vi "Word Find & Replace.vi"   [LabVIEW 2010, in "NI_ReportGenerationToolkit.lvlib"]
doc: "Finds and replaces a text segment. The data type you wire to the <B>replace with</B> input determines the polymorphic instance to use."
uses:
  <vilib>/addons/_office/NI_ReportGenerationToolkit.lvlib
  <vilib>/Utility/NIReport.llb/Word/NI_Word.lvclass
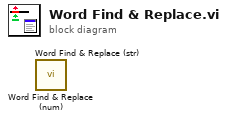
[diagram p0: block diagram]
diagram:
  n1 = call <vilib>:"Word Find & Replace (num).vi"() -> ()  [unwired: 13 in, 3 out]
  n2 = call "Word Find & Replace (str).vi"() -> ()  [unwired: 13 in, 3 out]
